vi "SetSystemDefinitionPropertyValue_I32.vi"(8 "error in (no error)":errorcluster, 9 "value":i32, 10 "property name":string, 11 "BaseNodeType in":refnum<k24>) -> (0 "error out":errorcluster, 3 "BaseNodeType out":refnum<k24>)   [LabVIEW 2015, in "VeriStandTestUtilities.lvlib"]
uses:
  VeriStandTestUtilities.lvlib
  NationalInstruments.VeriStand.SystemStorage
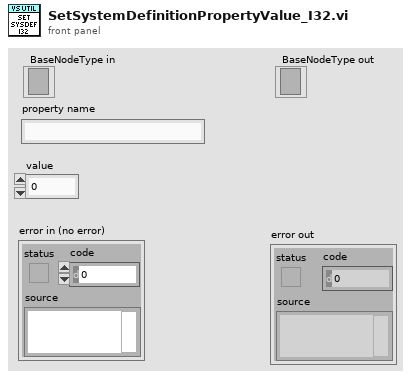
[diagram p1: front panel]
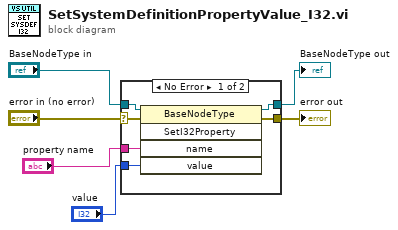
[diagram p0: block diagram]
diagram:
  n1 = case shown="No Error" "error in (no error)" {
    selector: "error in (no error)" -> [w11 w14]
    tunnel: "BaseNodeType in" -> [w12 w13]
    tunnel: "value" -> [w10 _]
    tunnel: "property name" -> [w9 _]
    tunnel: [w8 w13] -> w2
    tunnel: [w7 w14] -> w1
    frame No Error {
      n2 = invoke class="BaseNodeType" method="SetI32Property"(reference=w12, error in=w11, "name"=w9, "value"=w10) -> (reference out=w8:refnum<k24>, error out=w7:errorcluster)  [unwired: 1 in, 3 out]
    }
    frame Error {
    }
  }
  "error out" <- w1
  "BaseNodeType out" <- w2
